vi "Read from Hardware.vi"(8 "error in":errorcluster, 10 "values in":dbl[](array[numeric]), 11 "Rx execution unit in":refnum<class "Rx Execution Unit.lvclass">) -> (0 "error out":errorcluster, 2 "values out":dbl[](array[numeric]), 3 "Rx execution unit out":refnum<class "Rx Execution Unit.lvclass">)   [LabVIEW 2020, in "Ballard MIL-STD-1553 Engine.lvlib" / "Implementation.lvlib" / "Rx Execution Unit.lvclass"]
uses:
  Rx Execution Unit.lvclass
  C:/Users/nitest/Desktop/Git 2020/niveristand-aim-milStd1553-custom-device/Source/Custom Device Support/Engine/Implementation/Execution Unit/Execution Unit.lvclass
  Rx Execution Unit.lvclass/Rx Execution Unit.ctl
  Custom Device/Write Error to System Log.vi/ca55ed61-c1f5-4d13-8aef-490b87d2cf89.vi
  <vilib>/NI VeriStand/Custom Device Tools/Custom Device Utility Library/NI VeriStand - Print Debug Line.vi
  Execution Unit/Execution Unit.lvclass
  Custom Device/Custom Device.lvlib
  <instrlib>/BTI1553Lib/BTI1553LV.lvlib
  <instrlib>/BTI1553Lib/Public/Controls/1553 Message Fields.ctl
  C:/Users/nitest/Desktop/Git 2020/niveristand-aim-milStd1553-custom-device/Source/Custom Device Support/Engine/Interfaces/Execution Unit/Execution Unit.lvclass
  C:/Users/nitest/Desktop/Git 2020/niveristand-aim-milStd1553-custom-device/Source/Custom Device Support/Engine/Implementation/Rx Execution Unit/Rx Execution Unit.lvclass
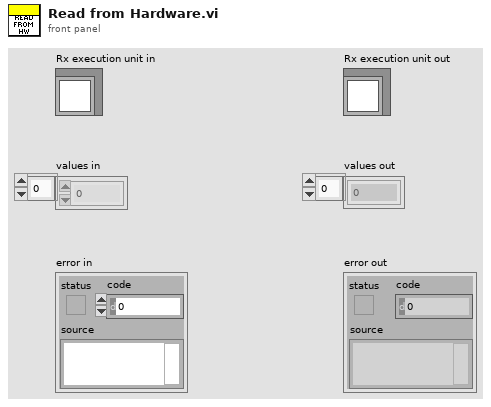
[diagram p1: front panel]
types:
  T1 = typedef "Ballard MIL-STD-1553 Engine.lvlib/Custom Device.lvlib/Hardware Handles.ctl" = cluster{"core handle":u64, "core reader handle":u64, "channel handles":u64[]}
  T2 = typedef "Rx Read Info.ctl" = cluster{"transfer handle":u64, "terminal address":u16}
  T3 = cluster{"core reader handle":u64, "core handle":u64}
  T4 = enum16{"unknown", "BC Message Buffer", "RT Message Buffer"}
  T5 = typedef "BTI1553LV.lvlib/1553 Message Fields.ctl" = cluster{"msgflag":u16, "msgopt":u16, "anyerror":bool, "noresponse":bool, "allretriesfailed":bool, "protocolerror":bool, "wrongsyncerror":bool, "datacounterror":bool, "manchestererror":bool, "parityerror":bool, "worderror":bool, "systemerror":bool, "hit":bool, "reserved":u8, "channelnumber":i32, "transmittedcwd1":bool, "transmittedcwd2":bool, "transmittedswd1":bool, "transmittedswd2":bool, "receivedcwd1":bool, "receivedcwd2":bool, "receivedswd1":bool, "receivedswd2":bool, "transmitteddwd":bool, "receiveddwd":bool, "reserved":i8, "reserved":i8, "bus":u32, "resptime1":u16, "resptime2":u16, "datacount":u16, "extflag":u16, "timetagh":u32, "timetag_hitcount":u32, "elapsetime_mintime_maxtime":u32, "cwd1":u16, "cwd2":u16, "swd1":u16, "swd2":u16, "data":u16[], "extra":u16[]}
  T6 = typedef "Ballard MIL-STD-1553 Engine.lvlib/Implementation.lvlib/Rx Execution Unit.lvclass/Status Error Counts.ctl" = cluster{"general protocol error count":u64, "improper number of words error count":u64, "manchester error count":u64, "monitor error count":u64, "parity error count":u64, "unconfigured frames error count":u64, "word error count":u64, "wrong sync error count":u64}
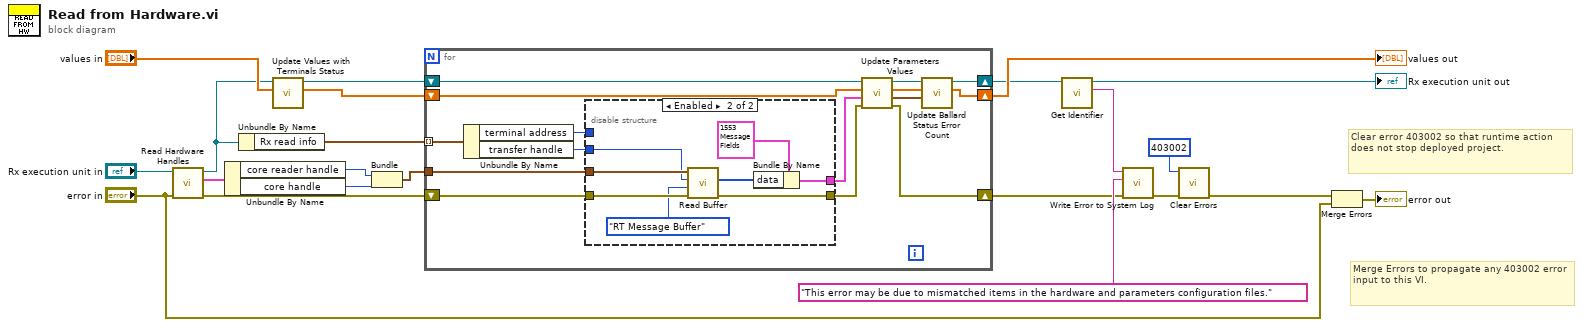
[diagram p0: block diagram]
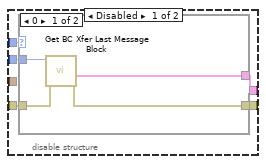
[diagram p2: hidden frame]
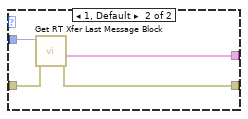
[diagram p3: hidden frame]
diagram:
  # "Clear error 403002 so that runtime action does not stop deployed project."
  # "Merge Errors to propagate any 403002 error input to this VI."
  n1 = call "Read Hardware Handles.vi"("error in"="error in", "Execution Unit in"="Rx execution unit in") -> ("error out"=w6:errorcluster, "hardware handles"=w4:T1, "Execution Unit out"=w8:refnum<class "Rx Execution Unit.lvclass">)  [unwired: 7 in]
  n2 = Unbundle By Name(w4) -> ("core reader handle"=w3:u64, "core handle"=w2:u64)
  n3 = Unbundle By Name(w8) -> ("Rx read info"=w5:T2[])
  n4 = call "Update Values with Terminals Status.vi"("values in"="values in", "Rx execution unit in"=w8) -> ("values out"=w10:dbl[], "Rx execution unit out"=w11:refnum<class "Rx Execution Unit.lvclass">)  [unwired: 7 in, 1 out]
  n5 = Bundle("core reader handle"=w3, "core handle"=w2) -> (w1:T3)  [unwired: 1 in]
  n6 = for {
    shift-right: [w30] -> w7
    shift-left: w6 -> [w25]
    shift-right: [w35] -> w22
    shift-left: w10 -> [w37]
    shift-right: [w36] -> w9
    shift-left: w11 -> [w32]
    tunnel: w5 -> [w24] mode=indexing
    tunnel: w1 -> [w23]
    n7 = Unbundle By Name(w24) -> ("terminal address"=w29:u16, "transfer handle"=w28:u64)
    n8 = disable-structure shown="Enabled" {
      disable-tunnel: w29 -> [w42 _]
      disable-tunnel: w28 -> [w41 w54]
      disable-tunnel: [w40 w53] -> w27
      disable-tunnel: [w39 w57] -> w26
      disable-tunnel: w25 -> [w38 w58]
      disable-tunnel: w23 -> [_ w55]
      frame Disabled {
        n9 = case shown="0" w42 {
          tunnel: w41 -> [w45 w50]
          tunnel: w38 -> [w46 w49]
          tunnel: [w44 w47] -> w39
          tunnel: [w43 w48] -> w40
          frame 0 {
            n10 = call <instrlib>:"Get BC Xfer Last Message Block.vi"("error in (no error)"=w46, "bc transfer handle in"=w45) -> ("error out"=w44:errorcluster, "message fields out"=w43:T5)  [unwired: 6 in, 2 out]
          }
          frame 1, Default {
            n11 = call <instrlib>:"Get RT Xfer Last Message Block.vi"("error in (no error)"=w49, "rt transfer handle in"=w50) -> ("error out"=w47:errorcluster, "message fields out"=w48:T5)  [unwired: 6 in, 2 out]
          }
        }
      }
      frame Enabled {
        n12 = call "Read Buffer.vi"("Error In"=w58, "Buffer Type"=T4."RT Message Buffer" ("Buffer Type (BC)"), "Buffer ID"=w54, "Module Reference"=w55) -> ("Error Out"=w57:errorcluster, "Data Array Out"=w51:u16[])  [unwired: 4 in, 2 out]
        n13 = Bundle By Name(cluster=T5 {"msgflag"=0, "msgopt"=0, "anyerror"=FALSE, "noresponse"=FALSE, "allretriesfailed"=FALSE, "protocolerror"=FALSE, "wrongsyncerror"=FALSE, "datacounterror"=FALSE, "manchestererror"=FALSE, "parityerror"=FALSE, "worderror"=FALSE, "systemerror"=FALSE, "hit"=FALSE, "reserved"=0, "channelnumber"=0, "transmittedcwd1"=FALSE, "transmittedcwd2"=FALSE, "transmittedswd1"=FALSE, "transmittedswd2"=FALSE, "receivedcwd1"=FALSE, "receivedcwd2"=FALSE, "receivedswd1"=FALSE, "receivedswd2"=FALSE, "transmitteddwd"=FALSE, "receiveddwd"=FALSE, "reserved"=0, "reserved"=0, "bus"=0, "resptime1"=0, "resptime2"=0, "datacount"=0, "extflag"=0, "timetagh"=0, "timetag_hitcount"=0, "elapsetime_mintime_maxtime"=0, "cwd1"=0, "cwd2"=0, "swd1"=0, "swd2"=0, "data"=[], "extra"=[]} ("message fields"), "data"=w51) -> (w53:T5)
      }
    }
    n14 = call "Update Parameters Values.vi"("error in"=w26, "message fields"=w27, "values in"=w37, "Rx execution unit in"=w32) -> ("error out"=w30:errorcluster, "status error counts"=w34:T6, "values out"=w33:dbl[], "Rx execution unit out"=w31:refnum<class "Rx Execution Unit.lvclass">)  [unwired: 4 in]
    n15 = call "Update Ballard Status Error Count.vi"("status error counts"=w34, "values in"=w33, "Rx execution unit in"=w31) -> ("values out"=w35:dbl[], "Rx execution unit out"=w36:refnum<class "Rx Execution Unit.lvclass">)  [unwired: 7 in]
  }
  "values out" <- w22
  n16 = call-dynamic "Get Identifier.vi"("Execution Unit Implementation in"=w9) -> ("Identifier"=w16:string, "Execution Unit Implementation out"=→"Rx execution unit out":refnum<class "Rx Execution Unit.lvclass">)  [unwired: 8 in, 1 out]
  n17 = call "Write Error to System Log.vi"("error in"=w7, "message"="This error may be due to mismatched items in the hardware and parameters configuration files.", "identifier"=w16) -> ("error out"=w15:errorcluster)  [unwired: 8 in]
  n18 = call <vilib>:"Clear Errors.vi"("error in (no error)"=w15, "specific error code to clear (0: all)"=403002) -> ("error out"=w18:errorcluster)  [unwired: 4 in, 1 out]
  n19 = Merge Errors(w18, "error in") -> (→"error out":errorcluster)
